vi "Write setup configuration.vi"(8 "error in (no error)":errorcluster, 11 "Channel in":refnum<class "Channel.lvclass">) -> (0 "error out":errorcluster, 3 "Channel out":refnum<class "Channel.lvclass">)   [LabVIEW 2018, in "Channel.lvclass"]
uses:
  Channel.lvclass
  Channel.lvclass/Channel.ctl
  Simulated_CCD_Camera/Simulated Camera.lvclass/Simulated Camera.ctl
  Simulated_CCD_Camera/Simulated Camera.lvclass
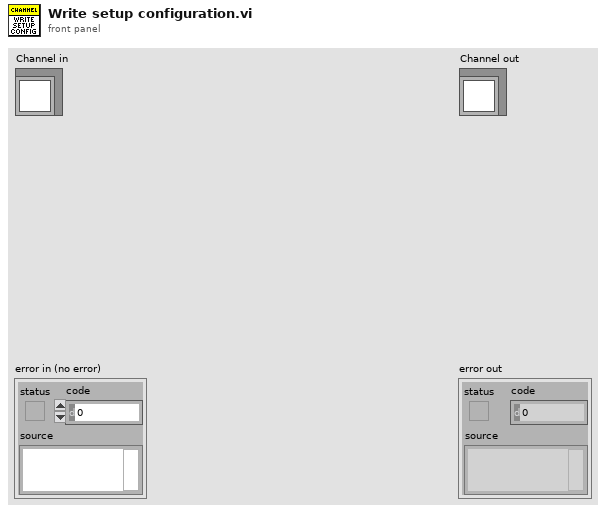
[diagram p1: front panel]
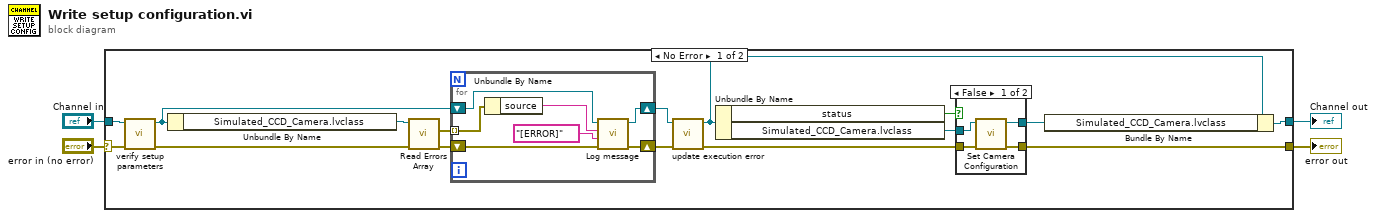
[diagram p0: block diagram]
diagram:
  n1 = case shown="No Error" "error in (no error)" {
    selector: "error in (no error)" -> [w15 w35]
    tunnel: [w19 w35] -> w3
    tunnel: [w17 w34] -> w1
    tunnel: "Channel in" -> [w16 w34]
    frame No Error {
      n2 = call "verify setup parameters.vi"("error in (no error)"=w15, "Channel in"=w16) -> ("error out"=w6:errorcluster, "Channel out"=w8:refnum<class "Channel.lvclass">)  [unwired: 8 in]
      n3 = Unbundle By Name(w8) -> ("Simulated_CCD_Camera.lvclass"=w9:refnum<class "Simulated Camera.lvclass">)
      n4 = call "Read Errors Array.vi"("error in (no error)"=w6, "Simulated_CCD_Camera in"=w9) -> ("error out"=w11:errorcluster, "Errors array"=w10:errorcluster[])  [unwired: 7 in, 1 out]
      n5 = for {
        shift-right: [w26] -> w13
        shift-left: w8 -> [w27]
        shift-right: [w25] -> w12
        shift-left: w11 -> [w23]
        tunnel: w10 -> [w22] mode=indexing
        n6 = Unbundle By Name(w22) -> ("source"=w21:string)
        n7 = call "Log message.vi"("error in (no error)"=w23, "message type"="[ERROR]", "String"=w21, "Channel in"=w27) -> ("error out"=w25:errorcluster, "Channel out"=w26:refnum<class "Channel.lvclass">)  [unwired: 6 in]
      }
      n8 = call "update execution error.vi"("error in (no error)"=w12, "Channel in"=w13) -> ("error out"=w5:errorcluster, "Channel out"=w7:refnum<class "Channel.lvclass">)  [unwired: 8 in]
      n9 = Unbundle By Name(w7) -> ("status"=w14:bool, "Simulated_CCD_Camera.lvclass"=w20:refnum<class "Simulated Camera.lvclass">)
      n10 = case shown="False" w14 {
        tunnel: w20 -> [w31 w33]
        tunnel: w5 -> [w30 w32]
        tunnel: [w28 w32] -> w19
        tunnel: [w29 w33] -> w18
        frame False {
          n11 = call-dynamic "Set Camera Configuration.vi"("error in (no error)"=w30, "CCDCamera in"=w31) -> ("error out"=w28:errorcluster, "CCDCamera out"=w29:refnum<class "Simulated Camera.lvclass">)  [unwired: 8 in]
        }
        frame True {
        }
      }
      n12 = Bundle By Name(cluster=w7, "Simulated_CCD_Camera.lvclass"=w18) -> (w17:refnum<class "Channel.lvclass">)
    }
    frame Error {
    }
  }
  "error out" <- w3
  "Channel out" <- w1
